vi "Cleanup When BD.vi"(8 "error in (no error)":errorcluster, 11 "VI in":refnum<vi>) -> (0 "error out":errorcluster, 3 "VI out":refnum<vi>)   [LabVIEW 2020, in "Mock Class Generator.lvclass"]
uses:
  Mock Class Generator.lvclass
  <vilib>/Utility/traverseref.llb/TRef TravTarget.ctl
  Mock Class Generator.lvclass/Mock Class Generator.ctl
  <vilib>/Utility/traverseref.llb/VI Scripting - Traverse.lvlib
panel:
  out "Array":string[](array[string])
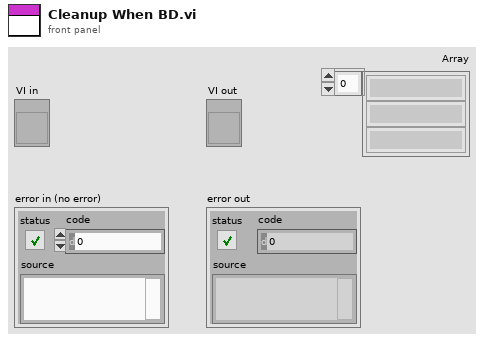
[diagram p1: front panel]
types:
  T1 = typedef "TRef TravTarget.ctl" = enum16{"FP", "BD", "Other"}
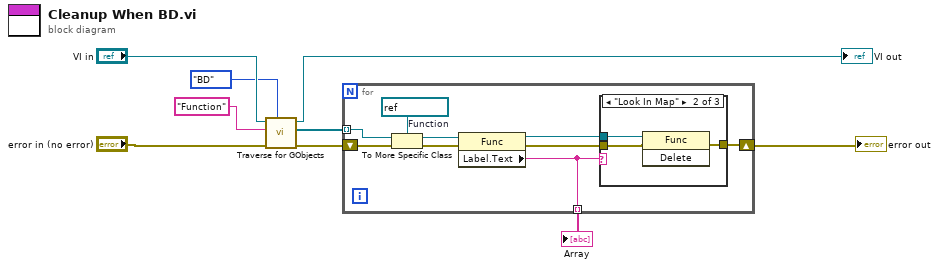
[diagram p0: block diagram]
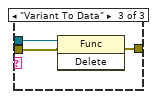
[diagram p3: hidden frame]
diagram:
  n1 = call <vilib>:"Traverse for GObjects.vi"("Traverse Target"=TRef_TravTarget."BD", "error in (no error)"="error in (no error)", "Class Name"="Function" ("name/order"), "VI Refnum"="VI in") -> ("error out"=w6:errorcluster, "References"=w5:refnum<vi>[], "dup VI Refnum"=→"VI out":refnum<vi>)  [unwired: 4 in, 1 out]
  n2 = for {
    tunnel: w5 -> [w12] mode=indexing
    shift-right: [w18] -> w3
    shift-left: w6 -> [w17]
    tunnel: [w14] -> w1 mode=indexing
    w10 = refnum<vi> refnum  # Function
    n3 = To More Specific Class(target class=w10, reference=w12, error in=w17) -> (specific class reference=w11:refnum<vi>, error out=w13:errorcluster)
    n4 = property class="Func"(reference=w11, error in=w13) -> (reference out=w15:refnum<vi>, error out=w16:errorcluster, "Label.Text"=w14:string)
    n5 = case shown="\"Look In Map\"" w14 {
      tunnel: [w19 w22 w25] -> w18
      tunnel: w16 -> [w19 w21 w24]
      tunnel: w15 -> [_ w20 w23]
      frame Default {
      }
      frame "Look In Map" {
        n6 = invoke class="Func" method="Delete"(reference=w20, error in=w21) -> (error out=w22:errorcluster)  [unwired: 1 in, 2 out]
      }
      frame "Variant To Data" {
        n7 = invoke class="Func" method="Delete"(reference=w23, error in=w24) -> (error out=w25:errorcluster)  [unwired: 1 in, 2 out]
      }
    }
  }
  "error out" <- w3
  "Array" <- w1
